vi "test Loopback Deployment.vi"(8 "error in":errorcluster, 11 "reference in":refnum<class "AIM_Deployment.lvclass">) -> (0 "error out":errorcluster, 3 "reference out":refnum<class "AIM_Deployment.lvclass">)   [LabVIEW 2020, in "AIM_Deployment.lvclass"]
uses:
  AIM_Deployment.lvclass
  AIM_Deployment.lvclass/AIM_Deployment.ctl
  b396e5f9-bef9-40c7-8d06-c3a1c8b08d2b.vi
  <vilib>/addons/_JKI Toolkits/VI Tester/TestCase.llb/TestCase.lvclass
  C:/Program Files (x86)/National Instruments/LabVIEW 2020/vi.lib/addons/_JKI Toolkits/VI Tester/TestCase.llb/TestCase.lvclass
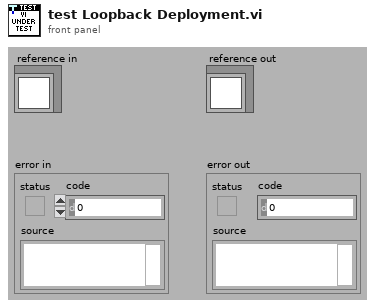
[diagram p1: front panel]
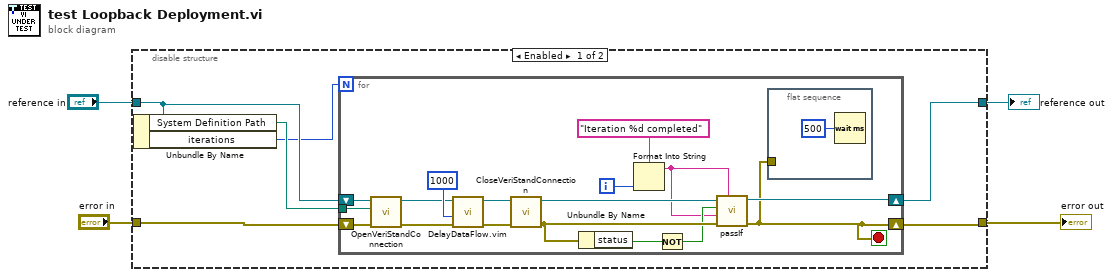
[diagram p0: block diagram]
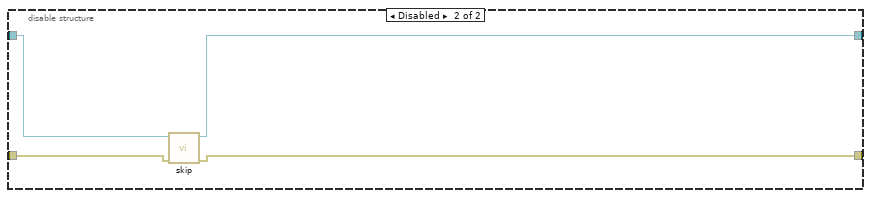
[diagram p2: hidden frame]
diagram:
  n1 = disable-structure shown="Enabled" {
    disable-tunnel: "reference in" -> [w10 w31]
    disable-tunnel: "error in" -> [w9 w30]
    disable-tunnel: [w8 w29] -> w2
    disable-tunnel: [w6 w28] -> w1
    frame Enabled {
      n2 = Unbundle By Name(w10) -> ("System Definition Path"=w7:path, "iterations"=w5:i32)
      n3 = for {
        N: w5 -> [_]
        tunnel: w7 -> [w20]
        shift-right: [w15] -> w6
        shift-left: w10 -> [w24]
        shift-right: [w12] -> w8
        shift-left: w9 -> [w23]
        i -> [w14]
        stop <- w12 stop-if-true
        n4 = call-dynamic "OpenVeriStandConnection.vi"("error in (no error)"=w23, "System Definition File"=w20, "VeriStand Test Case in"=w24) -> ("error out"=w22:errorcluster, "VeriStand Test Case out"=w21:refnum<class "AIM_Deployment.lvclass">)  [unwired: 6 in, 1 out]
        n5 = call "DelayDataFlow.vim"("value in"=w22, "milliseconds to wait"=u32 1000) -> ("value out"=w26:errorcluster)  [unwired: 2 in, 1 out]
        n6 = call-dynamic "CloseVeriStandConnection.vi"("error in (no error)"=w26, "VeriStand Test Case in"=w21) -> ("error out"=w19:errorcluster, "VeriStand Test Case out"=w16:refnum<class "AIM_Deployment.lvclass">)  [unwired: 8 in]
        n7 = Unbundle By Name(w19) -> ("status"=w18:bool)
        n8 = Format Into String(format string="Iteration %d completed", w14) -> (resulting string=w11:string)  [unwired: 2 in, 1 out]
        n9 = Not(x=w18) -> (.not. x?=w17:bool)
        n10 = call-dynamic "passIf.vi"("custom report message (\"\")"=w11, "error in (no error)"=w19, "message (\"\")"=w11, "pass"=w17, "TestCase in"=w16) -> ("error out"=w12:errorcluster, "TestCase out"=w15:refnum<class "AIM_Deployment.lvclass">)  [unwired: 5 in]
        n11 = flat-sequence {
          tunnel: w12 -> [_]
          frame #0 {
            n12 = Wait (ms)(milliseconds to wait=u32 500) -> ()  [unwired: 1 out]
          }
        }
      }
    }
    frame Disabled {
      n13 = call <vilib>:"skip.vi"("error in (no error)"=w30, "TestCase in"=w31) -> ("error out"=w29:errorcluster, "TestCase out"=w28:refnum<class "AIM_Deployment.lvclass">)  [unwired: 8 in]
    }
  }
  "error out" <- w2
  "reference out" <- w1
